vi "Set Index.vi"(8 "error in (no error)":errorcluster, 10 "Index":i32, 11 "Vector in":refnum<class "Vector.lvclass">) -> (0 "error out":errorcluster, 3 "Vector out":refnum<class "Vector.lvclass">)   [LabVIEW 2021, in "Vector.lvclass"]
uses:
  Vector.lvclass
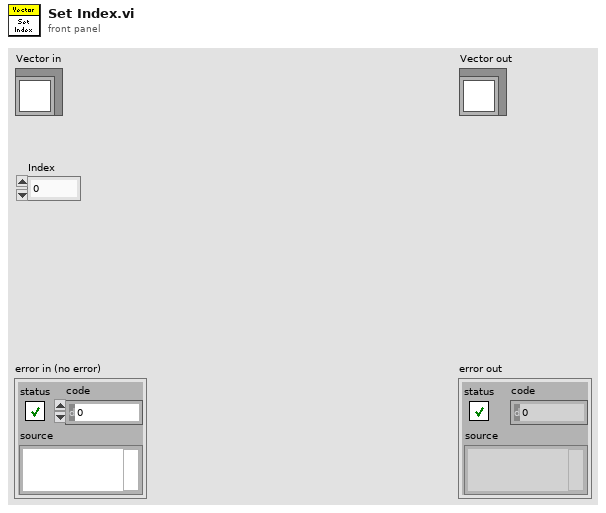
[diagram p1: front panel]
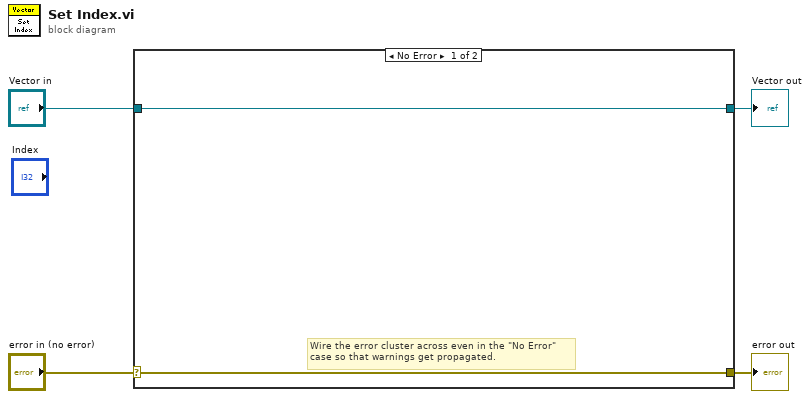
[diagram p0: block diagram]
diagram:
  n1 = case shown="No Error" "error in (no error)" {
    selector: "error in (no error)" -> [w5 w8]
    tunnel: [w5 w8] -> w3
    tunnel: [w6 w7] -> w1
    tunnel: "Vector in" -> [w6 w7]
    frame No Error {
      # "Wire the error cluster across even in the \"No Error\"\ncase so that warnings get propagated."
    }
    frame Error {
    }
  }
  "error out" <- w3
  "Vector out" <- w1
